vi "Save_subVi.vi"(8 "error in (no error)":errorcluster) -> (0 "error out":errorcluster)   [LabVIEW 2019]
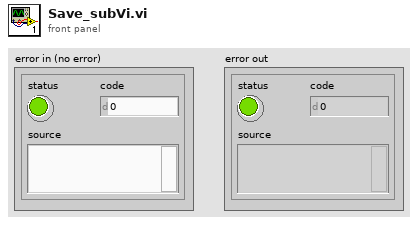
[diagram p1: front panel]
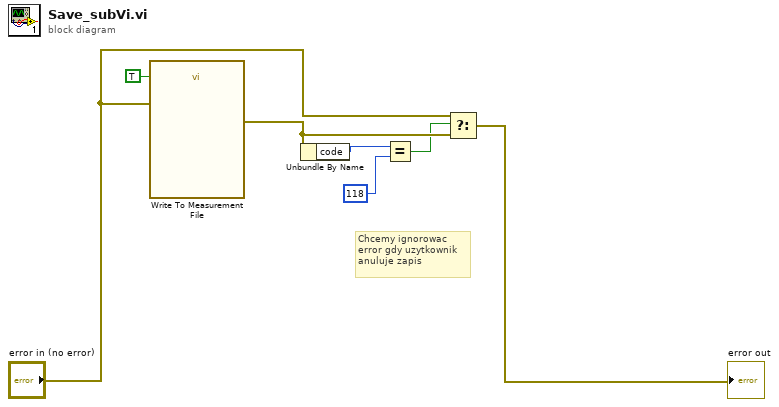
[diagram p0: block diagram]
diagram:
  # "Chcemy ignorowac\nerror gdy uzytkownik\nanuluje zapis"
  n1 = call "Write To Measurement File"("Reset"=TRUE, "error in (no error)"="error in (no error)") -> ("error out"=w5:errorcluster)  [unwired: 15 in, 2 out]
  n2 = Unbundle By Name(w5) -> ("code"=w2:i32)
  n3 = Equal?(x=w2, y=118) -> (x = y?=w4:bool)
  n4 = Select(t="error in (no error)", s=w4, f=w5) -> (s? t:f=→"error out":errorcluster)
